vi "validate_arguments.vi"(6 "vmin":refnum<vi>, 9 "upper time":refnum<vi>, 10 "lower time":refnum<vi>, 11 "vmax":refnum<vi>) -> (3 "Problem":bool, 4 "String":string)   [LabVIEW 2015]
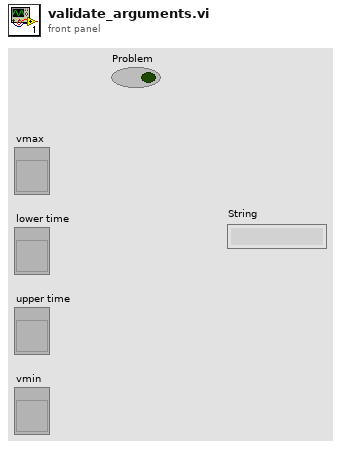
[diagram p1: front panel]
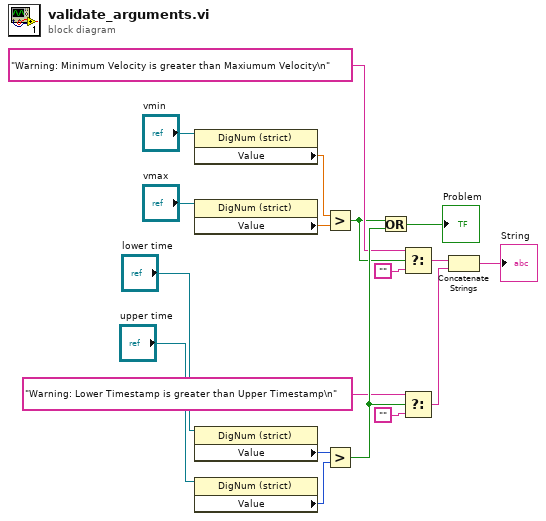
[diagram p0: block diagram]
diagram:
  n1 = property class="DigNum (strict)"(reference="vmin") -> ("Value"=w14:dbl)  [unwired: 1 in, 2 out]
  n2 = property class="DigNum (strict)"(reference="vmax") -> ("Value"=w13:dbl)  [unwired: 1 in, 2 out]
  n3 = property class="DigNum (strict)"(reference="lower time") -> ("Value"=w12:i64)  [unwired: 1 in, 2 out]
  n4 = property class="DigNum (strict)"(reference="upper time") -> ("Value"=w11:i64)  [unwired: 1 in, 2 out]
  n5 = Greater?(x=w14, y=w13) -> (0:w1:bool)
  n6 = Greater?(x=w12, y=w11) -> (0:w9:bool)
  n7 = Or(x=w1, y=w9) -> (x .or. y?=→"Problem":bool)
  n8 = Select(t="Warning: Minimum Velocity is greater than Maxiumum Velocity\n", s=w1, f="") -> (s? t:f=w4:string)
  n9 = Select(t="Warning: Lower Timestamp is greater than Upper Timestamp\n", s=w9, f="") -> (s? t:f=w3:string)
  n10 = Concatenate Strings(w4, w3) -> (→"String":string)
